vi "TDataProcess.vi"(1 "温度数组":dbl[](array[numeric])) -> (0 "温度值":dbl)   [LabVIEW 2012]
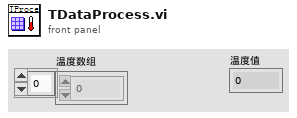
[diagram p1: front panel]
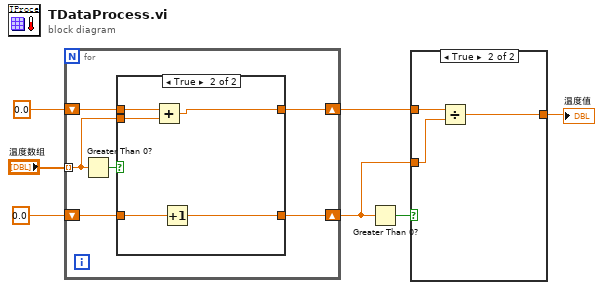
[diagram p0: block diagram]
diagram:
  n1 = for {
    tunnel: "温度数组" -> [w8] mode=indexing
    shift-right: [w11] -> w3
    shift-left: 0.0 -> [w12]
    shift-right: [w10] -> w2
    shift-left: 0.0 -> [w9]
    n2 = Greater Than 0?(x=w8) -> (x > 0?=w13:bool)
    n3 = case shown="True" w13 {
      tunnel: w12 -> [w15 w18]
      tunnel: [w15 w17] -> w11
      tunnel: [w14 w19] -> w10
      tunnel: w9 -> [w14 w20]
      tunnel: w8 -> [_ w16]
      frame False {
      }
      frame True {
        n4 = Add(x=w18, y=w16) -> (x+y=w17:dbl)
        n5 = Increment(x=w20) -> (x+1=w19:dbl)
      }
    }
  }
  n6 = Greater Than 0?(x=w2) -> (x > 0?=w4:bool)
  n7 = case shown="True" w4 {
    tunnel: w3 -> [_ w23]
    tunnel: w2 -> [_ w22]
    tunnel: [_ w21] -> w1
    frame False {
    }
    frame True {
      n8 = Divide(x=w23, y=w22) -> (x/y=w21:dbl)
    }
  }
  "温度值" <- w1
